vi "Frame Sync Test.vi"() -> ()   [LabVIEW 2013]
uses:
  <vilib>/Waveform/DWDTOps.llb/DWDT Boolean Array to Digital.vi
  <vilib>/Waveform/DWDTOps.llb/DWDT Append Digital Samples.vi
  <vilib>/Waveform/DWDTOps.llb/DWDT Digital to Binary U8.vi
  <vilib>/Waveform/DWDTOps.llb/DWDT Binary U8 to Digital.vi
  Source/I2S-TDM.lvlib
panel:
  in  "stop":bool
  in  "Pause":bool
  in  "milliseconds to wait":u32(slide)=10 scale=0.0..100.0
  out "Digital Waveform Graph":digitalwaveform(graph)
  in  "Graph Size":i32=100
  in  "channel count (2)":u8=2
  in  "prev output valid":bool
  in  "data sample edge (rising)":enum16{"rising", "falling"}(ring)
  in  "start delay (0)":u8
  in  "frame sync in":bool
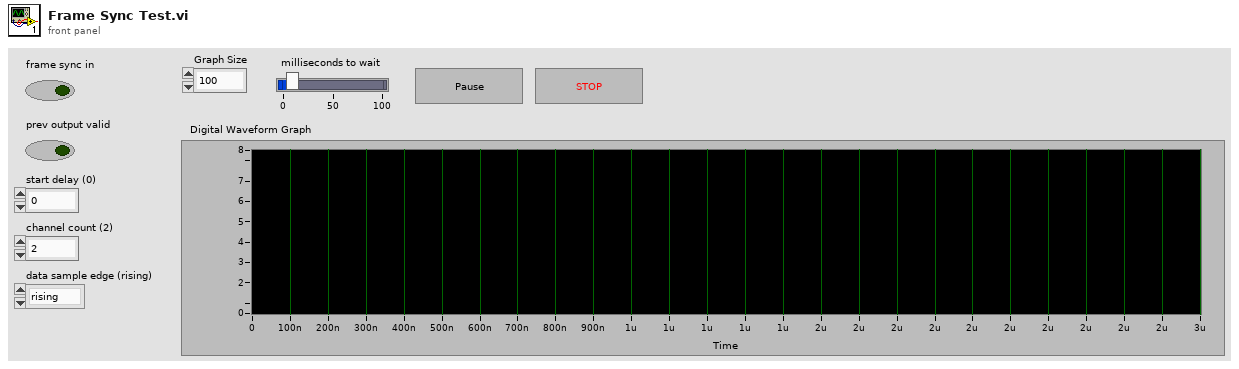
[diagram p1: front panel]
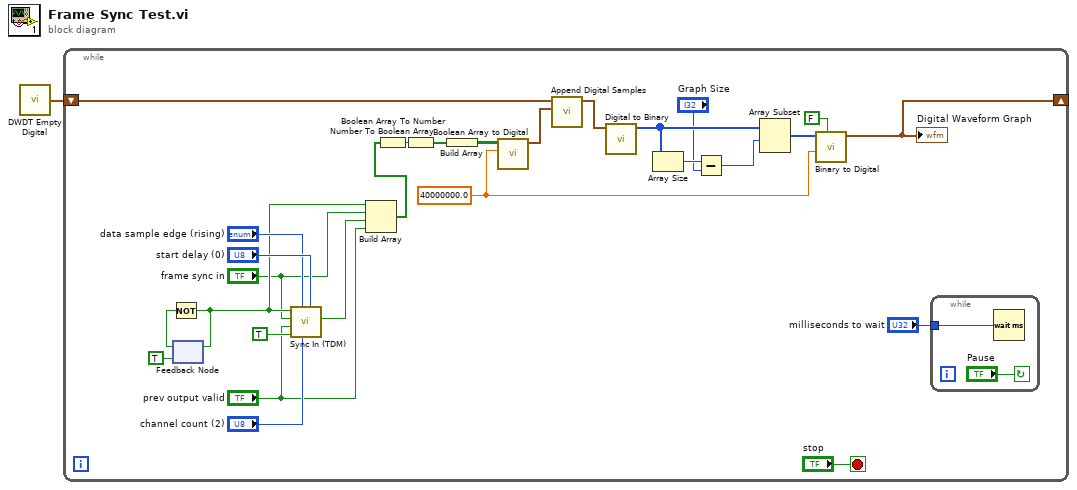
[diagram p0: block diagram]
diagram:
  n1 = call <vilib>:"DWDT Empty Digital.vi"() -> ("digital waveform out"=w1:digitalwaveform)  [unwired: 5 in]
  n2 = while {
    shift-right: [w9] -> _
    shift-left: w1 -> [w10]
    stop <- "stop" stop-if-true
    w15 = 40000000.0 ("sample rate")
    n3 = feedback #1(TRUE) -> (w28:bool)
    n4 = Not(x=w28) -> (.not. x?=w6:bool)
    n5 = feedback-in #1(w6) -> ()
    n6 = call "Sync In (TDM).vi"("start delay (0)"="start delay (0)", "channel count (2)"="channel count (2)", "data sample edge (rising)"="data sample edge (rising)", "receive"=TRUE, "prev transfer done"="prev output valid", "frame sync in"="frame sync in", "clock in"=w6) -> ("start read"=w3:bool)  [unwired: 2 in, 2 out]
    n7 = Build Array(w6, "frame sync in", w3, "prev output valid") -> (w4:bool[])
    n8 = Boolean Array To Number(Boolean array=w4) -> (number=w12:u8)
    n9 = Number To Boolean Array(number=w12) -> (Boolean array=w11:bool[])
    n10 = Build Array(w11) -> (w16:bool[][])
    n11 = call-poly <vilib>:"Boolean Array to Digital.vi"("sample rate"=w15, "boolean array"=w16) -> ("digital waveform"=w14:digitalwaveform)  [unwired: 8 in, 1 out]
    n12 = call-poly <vilib>:"Append Digital Samples.vi"("digital waveform B"=w14, "digital waveform A"=w10) -> ("digital waveform out"=w13:digitalwaveform)  [unwired: 8 in, 1 out]
    n13 = call-poly <vilib>:"Digital to Binary.vi"("digital waveform"=w13) -> ("binary array"=w22:u8[])  [unwired: 9 in, 1 out]
    n14 = Array Size(array=w22) -> (size(s)=w21:i32)
    n15 = Subtract(x=w21, y="Graph Size") -> (x-y=w20:i32)
    n16 = Array Subset(array=w22, index=w20) -> (w17:u8[])  [unwired: 1 in]
    n17 = call-poly <vilib>:"Binary to Digital.vi"("compress data (T)"=FALSE, "sample rate"=w15, "binary array"=w17) -> ("digital waveform"=w9:digitalwaveform)  [unwired: 7 in, 1 out]
    "Digital Waveform Graph" <- w9
    n18 = while {
      tunnel: "milliseconds to wait" -> [w29]
      stop <- "Pause" continue-if-true
      n19 = Wait (ms)(milliseconds to wait=w29) -> ()  [unwired: 1 out]
    }
  }
